vi "Configure Serial Bus (M1553 - Trigger).vi"(0 "VISA resource name":refnum<visa-resource-name>, 1 "Remote Terminal Address (0)":dbl, 5 "Serial Bus Name (1: Serial Bus 1)":i32(ring)=1 items=["Serial Bus 1"=1, "Serial Bus 2"=2], 9 "Trigger Type (2: CSTA)":i32(ring)=2 items=["Data Word Start", "Data Word Stop", "Command/Status Word Start", "Command/Status Word Stop", "RTA", "Parity Error", "Sync Error", "Manchester Error", "RTA11"], 11 "error in (no error)":errorcluster, 12 "Data Pattern (XXXXXXXXXXX)":string="XXXXXXXXXXX") -> (4 "VISA resource name out":refnum<visa-resource-name>, 15 "error out":errorcluster)   [LabVIEW 2017, in "Agilent 2000 3000 X-Series.lvlib"]
doc: "Configures the trigger settings of MIL- STD- 1553 bus.\n\nNote:\nThis VI is not supported by EDUX1052A/G, DSOX1202A/G, DSOX1204A/G models"
uses:
  Agilent 2000 3000 X-Series.lvlib
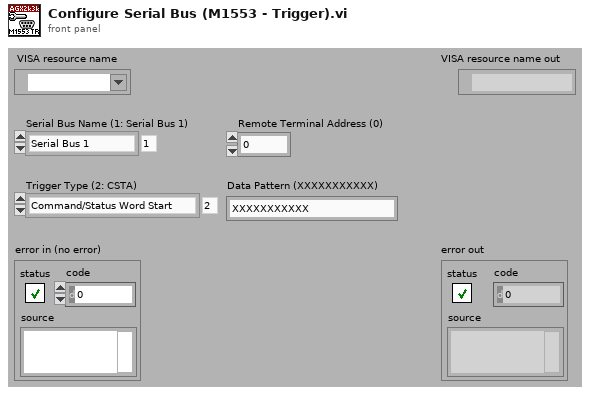
[diagram p1: front panel]
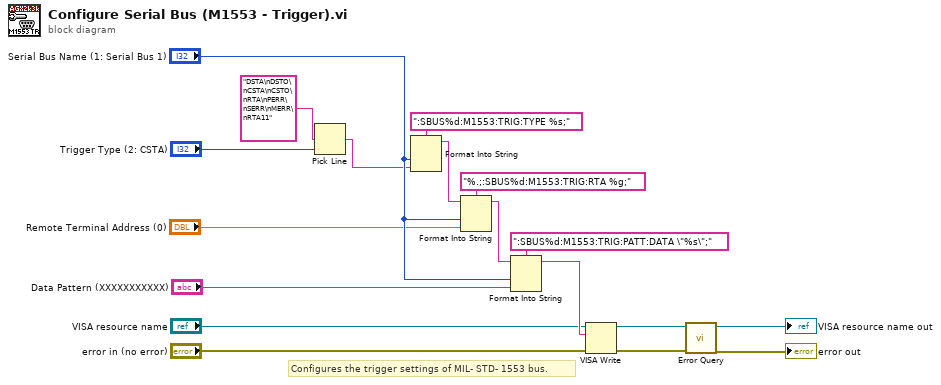
[diagram p0: block diagram]
diagram:
  # "Configures the trigger settings of MIL- STD- 1553 bus."
  n1 = Pick Line(multi-line string="DSTA\nDSTO\nCSTA\nCSTO\nRTA\nPERR\nSERR\nMERR\nRTA11", line index="Trigger Type (2: CSTA)") -> (output string=w14:string)  [unwired: 1 out]
  n2 = Format Into String(format string=":SBUS%d:M1553:TRIG:TYPE %s;", "Serial Bus Name (1: Serial Bus 1)", w14) -> (resulting string=w13:string)  [unwired: 2 in, 1 out]
  n3 = Format Into String(format string="%.;:SBUS%d:M1553:TRIG:RTA %g;", initial string=w13, "Serial Bus Name (1: Serial Bus 1)", "Remote Terminal Address (0)") -> (resulting string=w10:string)  [unwired: 1 in, 1 out]
  n4 = Format Into String(format string=":SBUS%d:M1553:TRIG:PATT:DATA \"%s\";", initial string=w10, "Serial Bus Name (1: Serial Bus 1)", "Data Pattern (XXXXXXXXXXX)") -> (resulting string=w7:string)  [unwired: 1 in, 1 out]
  n5 = VISA Write(VISA resource name="VISA resource name", write buffer=w7, error in (no error)="error in (no error)") -> (VISA resource name out=w4:refnum<visa-resource-name>, error out=w3:errorcluster)  [unwired: 1 out]
  n6 = call "Error Query.vi"("error in (no error)"=w3, "VISA resource name"=w4) -> ("error out"=→"error out":errorcluster, "VISA resource name out"=→"VISA resource name out":refnum<visa-resource-name>)  [unwired: 8 out]
